vi "terminate.vi"(8 "error in (no error)":errorcluster, 11 "GenericPlugin in":refnum<class "FPGAWrapperMH120124RAPS_PXI7813R.lvclass">) -> (0 "error out":errorcluster, 3 "GenericPlugin out":refnum<class "FPGAWrapperMH120124RAPS_PXI7813R.lvclass">)   [LabVIEW 2010, in "FPGAWrapperMH120124RAPS_PXI7813R.lvclass"]
doc: "The dynamic dispatch version of this VI terminates the plug-in object by releasing all of its resources."
uses:
  FPGAWrapperMH120124RAPS_PXI7813R.lvclass
  class_data.vi
  grabber/command_enum.ctl
  common/classes/ErrorController/ErrorController/ErrorController.lvclass
  GenericFPGAWrapper/GenericFPGAWrapper/GenericFPGAWrapper.lvclass
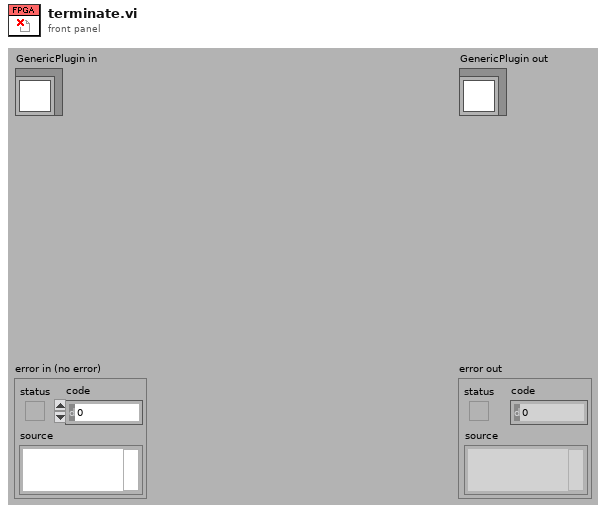
[diagram p1: front panel]
types:
  T1 = typedef "command_enum.ctl" = enum8{"NULL", "update", "start", "stop", "reset", "shut-down"}
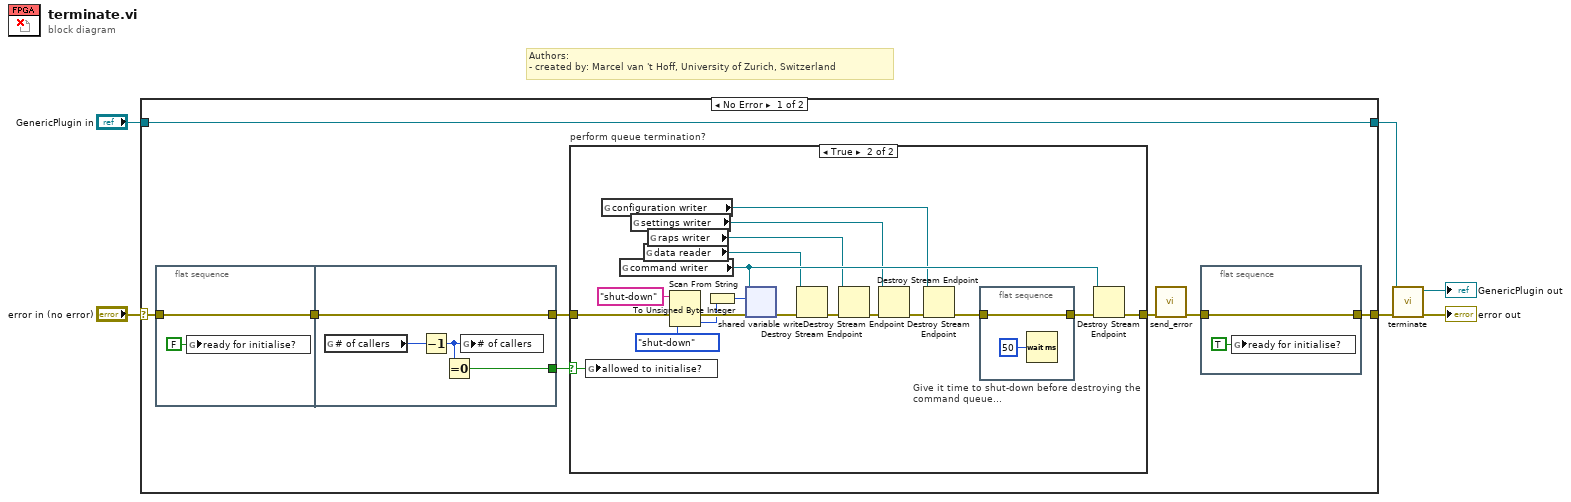
[diagram p0: block diagram]
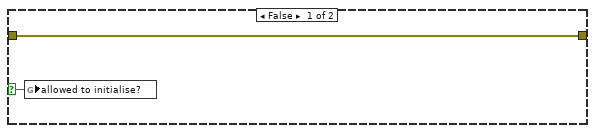
[diagram p2: hidden frame]
diagram:
  # "Authors: \n- created by: Marcel van 't Hoff, University of Zurich, Switzerland"
  n1 = case shown="No Error" "error in (no error)" {
    selector: "error in (no error)" -> [w12 w46]
    tunnel: "GenericPlugin in" -> [w14 w47]
    tunnel: [w14 w47] -> w1
    tunnel: [w7 w46] -> w2
    frame No Error {
      n2 = flat-sequence {
        tunnel: w12 -> [w17]
        tunnel: [w17] -> w11
        tunnel: [w20] -> w9
        tunnel: [w19] -> w10
        tunnel: w11 -> [w19]
        frame #0 {
          n3 = global write "class_data.vi" "ready for initialise?"(FALSE ("ready for initialise?")) -> ()
        }
        frame #1 {
          n4 = global read "class_data.vi" "# of callers"() -> (w22:i32)
          n5 = Decrement(x=w22) -> (x-1=w21:i32)
          n6 = Equal To 0?(x=w21) -> (x = 0?=w20:bool)
          n7 = global write "class_data.vi" "# of callers"(w21) -> ()
        }
      }
      n8 = case "perform queue termination?" shown="True" w9 {
        selector: w9 -> [w23 w26]
        tunnel: w10 -> [w24 w32]
        tunnel: [w24 w41] -> w13
        frame False {
          n9 = global write "class_data.vi" "allowed to initialise?"(w23) -> ()
        }
        frame True {
          n10 = global write "class_data.vi" "allowed to initialise?"(w26) -> ()
          n11 = global read "class_data.vi" "configuration writer"() -> (w35:refnum<k21>)
          n12 = global read "class_data.vi" "command writer"() -> (w39:refnum<k21>)
          n13 = global read "class_data.vi" "settings writer"() -> (w36:refnum<k21>)
          n14 = global read "class_data.vi" "data reader"() -> (w38:refnum<k21>)
          n15 = global read "class_data.vi" "raps writer"() -> (w37:refnum<k21>)
          n16 = Scan From String(input string="shut-down" ("format string"), error in=w32, default 1=command_enum."shut-down" ("command")) -> (error out=w31:errorcluster, output 1=w29:T1)  [unwired: 2 in, 2 out]
          n17 = To Unsigned Byte Integer(number=w29) -> (unsigned 8bit integer=w43:u8)
          n18 = shared-variable-write(w39, w31, w43) -> (w27:errorcluster)  [unwired: 1 in, 2 out]
          n19 = Destroy Stream Endpoint(8:w27, 11:w38) -> (0:w25:errorcluster)
          n20 = Destroy Stream Endpoint(8:w25, 11:w37) -> (0:w40:errorcluster)
          n21 = Destroy Stream Endpoint(8:w40, 11:w36) -> (0:w34:errorcluster)
          n22 = Destroy Stream Endpoint(8:w34, 11:w35) -> (0:w33:errorcluster)
          n23 = flat-sequence "Give it time to shut-down before destroying the command queue..." {
            tunnel: [w44] -> w42
            tunnel: w33 -> [w44]
            frame #0 {
              n24 = Wait (ms)(milliseconds to wait=u32 50) -> ()  [unwired: 1 out]
            }
          }
          n25 = Destroy Stream Endpoint(8:w42, 11:w39) -> (0:w41:errorcluster)
        }
      }
      n26 = call "send_error.vi"("error in (no error)"=w13) -> ("error out"=w8:errorcluster)  [unwired: 10 in]
      n27 = flat-sequence {
        tunnel: w8 -> [w15]
        tunnel: [w15] -> w7
        frame #0 {
          n28 = global write "class_data.vi" "ready for initialise?"(TRUE ("ready for initialise?")) -> ()
        }
      }
    }
    frame Error {
    }
  }
  n29 = call-parent "terminate.vi"("error in (no error)"=w2, "GenericPlugin in"=w1) -> ("error out"=→"error out":errorcluster, "GenericPlugin out"=→"GenericPlugin out":refnum<class "FPGAWrapperMH120124RAPS_PXI7813R.lvclass">)  [unwired: 8 in]
